vi "sequ.vi"   [LabVIEW 2019]
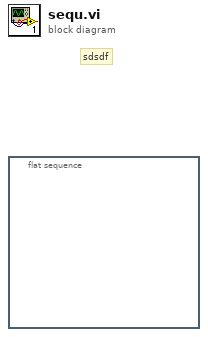
[diagram p0: block diagram]
diagram:
  # "sdsdf"
  n1 = flat-sequence {
    frame #0 {
    }
  }
